vi "Node.Settings.vi"(6 "Action":enum8{"Get", "Set"}(ring), 8 "error in (no error)":errorcluster, 10 "Node.Settings":T1 {"Name" format="%.0x"}, 11 "Item Ref in":T2 format="%.0x") -> (0 "error out":errorcluster, 2 "Node.Settings":T1 {"Name" format="%.0x"}, 3 "Item Ref out":T2 format="%.0x")   [LabVIEW 2019, in "J1939 Addon Shared.lvlib"]
uses:
  J1939 Addon Shared.lvlib
  <vilib>/NI VeriStand/Custom Device API/Custom Device Item Ref.ctl
  Types/Monitor Settings.ctl
  Constants.vi
  <vilib>/NI/NI VeriStand Advanced SysDef API/_SubVIs/SysDef.Property.Set.U32.vi
  <vilib>/NI/NI VeriStand Advanced SysDef API/_SubVIs/SysDef.Property.Set.String.vi
  <vilib>/NI/NI VeriStand Advanced SysDef API/_SubVIs/SysDef.Property.Set.Boolean.vi
  <vilib>/NI VeriStand/Custom Device API/Get Item Property (U32).vi
  <vilib>/NI VeriStand/Custom Device API/Get Item Property (String).vi
  <vilib>/NI VeriStand/Custom Device API/Get Item Property (Boolean).vi
  <vilib>/NI VeriStand/Custom Device API/Custom Device API.lvlib
  <vilib>/NI/NI VeriStand Advanced SysDef API/SysDef API/Advanced System Definition.lvlib
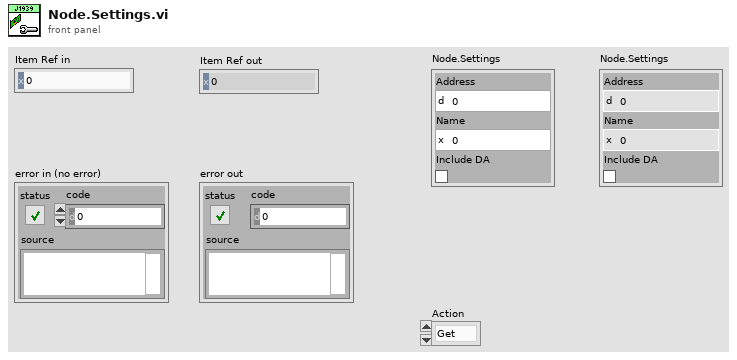
[diagram p1: front panel]
types:
  T1 = typedef "J1939 Addon Shared.lvlib/Monitor Settings.ctl" = cluster{"Address":u8, "Name":u64, "Include DA":bool}
  T2 = typedef "Custom Device API.lvlib/Custom Device Item Ref.ctl" = u64
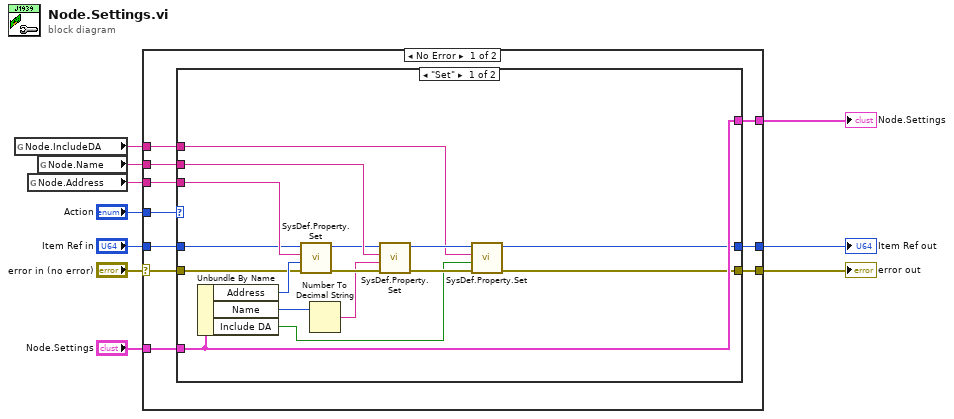
[diagram p0: block diagram]
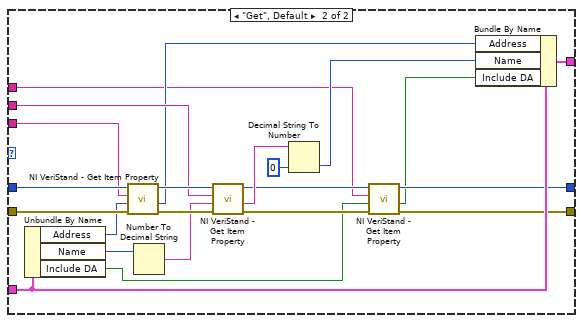
[diagram p2: hidden frame]
diagram:
  n1 = global read "Constants.vi" "Node.IncludeDA"() -> (w1:string)
  n2 = global read "Constants.vi" "Node.Address"() -> (w9:string)
  n3 = global read "Constants.vi" "Node.Name"() -> (w5:string)
  n4 = case shown="No Error" "error in (no error)" {
    selector: "error in (no error)" -> [w14 w60]
    tunnel: "Item Ref in" -> [w20 w59]
    tunnel: w9 -> [w19 _]
    tunnel: [w18 w60] -> w8
    tunnel: [w17 w59] -> w7
    tunnel: [w16 _] -> w6
    tunnel: w5 -> [w15 _]
    tunnel: "Node.Settings" -> [w13 _]
    tunnel: "Action" -> [w12 _]
    tunnel: w1 -> [w11 _]
    frame No Error {
      n5 = case shown="\"Set\"" w12 {
        tunnel: w20 -> [w33 w54]
        tunnel: w19 -> [w36 w50]
        tunnel: [w24 w41] -> w18
        tunnel: [w23 w40] -> w17
        tunnel: [w34 w58] -> w16
        tunnel: w15 -> [w35 w49]
        tunnel: w14 -> [w28 w55]
        tunnel: w13 -> [w34 w52]
        tunnel: w11 -> [w21 w39]
        frame "Set" {
          n6 = Unbundle By Name(w34) -> ("Address"=w30:u8, "Name"=w29:u64, "Include DA"=w22:bool)
          n7 = call-poly <vilib>:"SysDef.Property.Set.vi"("error in (no error)"=w28, "Value"=w30, "Property Name"=w36, "nodeID"=w33) -> ("error out"=w32:errorcluster, "nodeID out"=w31:u64)  [unwired: 6 in]
          n8 = Number To Decimal String(number=w29) -> (decimal integer string=w27:string)  [unwired: 1 in]
          n9 = call-poly <vilib>:"SysDef.Property.Set.vi"("error in (no error)"=w32, "Value"=w27, "Property Name"=w35, "nodeID"=w31) -> ("error out"=w25:errorcluster, "nodeID out"=w26:u64)  [unwired: 6 in]
          n10 = call-poly <vilib>:"SysDef.Property.Set.vi"("error in (no error)"=w25, "Value"=w22, "Property Name"=w21, "nodeID"=w26) -> ("error out"=w24:errorcluster, "nodeID out"=w23:u64)  [unwired: 6 in]
        }
        frame "Get", Default {
          n11 = Unbundle By Name(w52) -> ("Address"=w51:u8, "Name"=w53:u64, "Include DA"=w38:bool)
          n12 = call-poly <vilib>:"NI VeriStand - Get Item Property.vi"("error in (no error)"=w55, "Default Value"=w51, "Property Name"=w50, "Item Ref in"=w54) -> ("error out"=w57:errorcluster, "Value"=w47:u32, "Item Ref out"=w56:T2)  [unwired: 4 in, 1 out]
          n13 = Number To Decimal String(number=w53) -> (decimal integer string=w48:string)  [unwired: 1 in]
          n14 = call-poly <vilib>:"NI VeriStand - Get Item Property.vi"("error in (no error)"=w57, "Default Value"=w48, "Property Name"=w49, "Item Ref in"=w56) -> ("error out"=w42:errorcluster, "Value"=w46:string, "Item Ref out"=w43:T2)  [unwired: 4 in, 1 out]
          n15 = Decimal String To Number(string=w46, default (0L)=u64 0 ("default (0 I32)")) -> (number=w44:u64)  [unwired: 1 in, 1 out]
          n16 = call-poly <vilib>:"NI VeriStand - Get Item Property.vi"("error in (no error)"=w42, "Default Value"=w38, "Property Name"=w39, "Item Ref in"=w43) -> ("error out"=w41:errorcluster, "Value"=w37:bool, "Item Ref out"=w40:T2)  [unwired: 4 in, 1 out]
          n17 = Bundle By Name(cluster=w52, "Address"=w47, "Name"=w44, "Include DA"=w37) -> (w58:T1)
        }
      }
    }
    frame Error {
    }
  }
  "Item Ref out" <- w7
  "error out" <- w8
  "Node.Settings" <- w6
